vi "Type Write.vi"(4 "error in (no error)":errorcluster, 5 "Value":T2, 6 "Container State":T4, 7 "Display State In":T1) -> (0 "error out":errorcluster, 3 "Display State Out":T1)   [LabVIEW 2020, in "PXISlotGP.xctl"]
uses:
  PXISlotGP.xctl
  <vilib>/_xctls/Container State.ctl
  PXISlot XControl/Connector Type.ctl
  State.ctl
  AOAIRefs.ctl
  <vilib>/_xctls/XControlSupport.lvlib
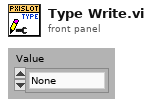
[diagram p1: front panel]
types:
  T1 = typedef "PXISlotGP.xctl/State.ctl" = cluster{"Connector Type":T2, "Hide unused":bool, "Trigger Visible":bool, "TabRef":refnum<vi>, "ConnRefs":refnum<vi>[], "PaneRef":refnum<vi>, "AOAIRefs":T3[], "TriggerRefs":refnum<vi>[], "check data":bool, "Name":string, "Events":cluster{"Type changed":refnum<user-event>}}
  T2 = typedef "Connector Type.ctl" = enum16{"None", "PXI-4461", "BNC-2110", "BNC-2090", "PXIe-4463", "PXIe-4464"}
  T3 = typedef "AOAIRefs.ctl" = cluster{"AORefs":refnum<vi>[], "AIRefs":refnum<vi>[]}
  T4 = typedef "XControlSupport.lvlib/Container State.ctl" = cluster{"Indicator?":bool, "Run Mode?":bool, " Refnum":refnum<vi>}
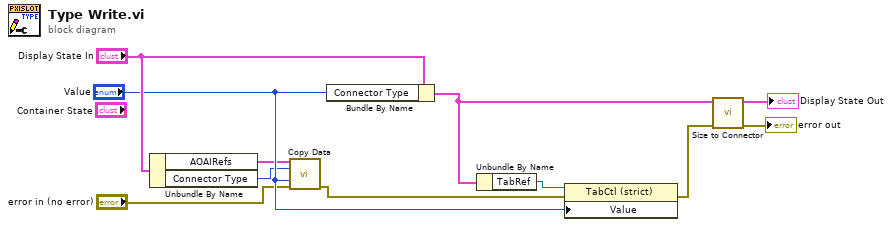
[diagram p0: block diagram]
diagram:
  n1 = Unbundle By Name("Display State In") -> ("AOAIRefs"=w4:T3[], "Connector Type"=w1:T2)
  n2 = call "Copy Data.vi"("AOAIRefs"=w4, "Old type"=w1, "New type"="Value", "error in (no error)"="error in (no error)") -> ("error out"=w2:errorcluster)  [unwired: 11 in]
  n3 = Bundle By Name(cluster="Display State In", "Connector Type"="Value") -> (w9:T1)
  n4 = Unbundle By Name(w9) -> ("TabRef"=w8:refnum<vi>)
  n5 = property class="TabCtl (strict)"(reference=w8, error in=w2, "Value"="Value") -> (error out=w7:errorcluster)  [unwired: 1 out]
  n6 = call "Size to Connector.vi"("error in (no error)"=w7, "Display State In in"=w9) -> ("error out"=→"error out":errorcluster, "Display State In out"=→"Display State Out":T1)  [unwired: 8 in]
